vi "X.1 Steering Encoder.vi"(1 "Steering Center":bool, 2 "Steer Encoder A":bool, 3 "Steer Encoder B":bool) -> (0 "Magic Number":i32)   [LabVIEW 2010]
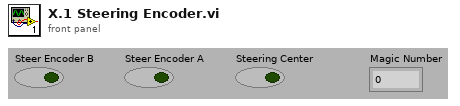
[diagram p1: front panel]
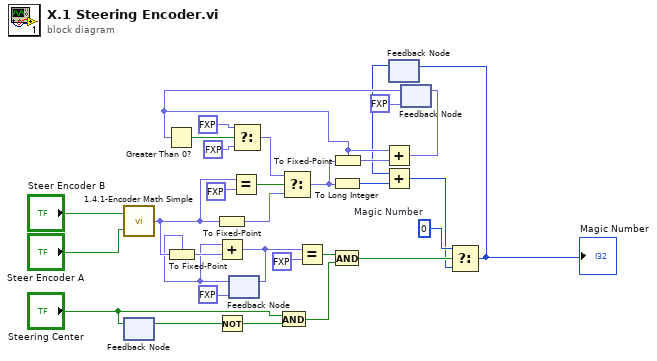
[diagram p0: block diagram]
diagram:
  w5 = 0  # Magic Number
  n1 = call "1.4.1-Encoder Math Simple.vi"("B"="Steer Encoder A", "A"="Steer Encoder B") -> ("Numeric"=w24:fxp<+/-,2,2>)
  n2 = feedback #1() -> (w7:bool)  [unwired: 1 in]
  n3 = feedback-in #1("Steering Center") -> ()
  n4 = To Fixed-Point(number=w24) -> (fixed-point=w25:fxp<+/-,3,3>)  [unwired: 1 in]
  n5 = Not(x=w7) -> (.not. x?=w6:bool)
  n6 = feedback #2(fxp<+/-,4,4> 0.0) -> (w8:fxp<+/-,4,4>)
  n7 = To Fixed-Point(fixed-point type=w8, number=w24) -> (fixed-point=w9:fxp<+/-,4,4>)
  n8 = Add(x=w8, y=w9) -> (x+y=w10:fxp<+/-,4,4>)
  n9 = feedback-in #2(w10) -> ()
  n10 = Equal?(x=w24, y=fxp<+/-,2,2> -2.0) -> (x = y?=w23:bool)
  n11 = And(x="Steering Center", y=w6) -> (x .and. y?=w12:bool)
  n12 = Equal?(x=w10, y=fxp<+/-,4,4> -8.0) -> (x = y?=w13:bool)
  n13 = And(x=w13, y=w12) -> (x .and. y?=w14:bool)
  n14 = feedback #3() -> (w1:i32)  [unwired: 1 in]
  n15 = feedback #4(fxp<+/-,3,3> 0.0) -> (w30:fxp<+/-,4,4>)
  n16 = Greater Than 0?(x=w30) -> (x > 0?=w31:bool)
  n17 = Select(t=fxp<+/-,3,3> 2.0 ("y"), s=w31, f=fxp<+/-,3,3> -2.0 ("y")) -> (s? t:f=w27:fxp<+/-,3,3>)
  n18 = Select(t=w27, s=w23, f=w25) -> (s? t:f=w26:fxp<+/-,3,3>)
  n19 = To Long Integer(number=w26) -> (32bit integer=w2:i32)
  n20 = To Fixed-Point(fixed-point type=w30, number=w26) -> (fixed-point=w21:fxp<+/-,4,4>)
  n21 = Add(x=w30, y=w21) -> (x+y=w20:fxp<+/-,4,4>)
  n22 = Add(x=w1, y=w2) -> (x+y=w4:i32)
  n23 = feedback-in #4(w20) -> ()
  n24 = Select(t=w5, s=w14, f=w4) -> (s? t:f=w3:i32)
  "Magic Number" <- w3
  n25 = feedback-in #3(w3) -> ()
